vi "lamquenmatran.vi"() -> ()   [LabVIEW 2019]
uses:
  <vilib>/Analysis/Matrix/Datatypes/RealMatrix.ctl
  <vilib>/Platform/TimedLoop/XDataNode/timing_clust.ctl
  <vilib>/Platform/TimedLoop/XDataNode/nitl_modes.ctl
  <vilib>/Platform/TimedLoop/XDataNode/wakeup.ctl
  <vilib>/Analysis/Matrix/Numeric/Conversions/Matrix To Array - RM.vi
  <vilib>/imath/engines/lvmath2/RunTimeEngine/BuiltInFunctions/is_empty/NIMS_is_empty(GM).vi
  <instcachedir>/0/NIMS_is_empty(GM)_AF8F13F4B7FD436CB1855477E2504B8A.lvgen/NIMS_is_empty(GM)_AF8F13F4B7FD436CB1855477E2504B8A_004.vi
  <vilib>/imath/engines/lvmath2/RunTimeEngine/ArithmeticOperatorToken/NIMS_ArithmeticOperator_multmx(M,CV)-internal.vi
  <instcachedir>/0/NIMS_ArithmeticOperator_multmx(M,CV)-internal_2C55777844884EEDB828A940D397C7D0.lvgen/NIMS_ArithmeticOperator_multmx(M,CV)-internal_2C55777844884EEDB828A940D397C7D0_001.vi
  <vilib>/imathl/engines/lvmath/Functions/Error Handling/Create Error.vi
  <vilib>/imath/engines/lvmath2/RunTimeEngine/IndexRead/NIMS V(S).vi
  <instcachedir>/0/NIMS V(S)_0488751826AF41519A22953C041130DC.lvgen/NIMS V(S)_0488751826AF41519A22953C041130DC_000.vi
  <vilib>/imath/engines/lvmath2/RunTimeEngine/ArithmeticOperatorToken/NIMS_ArithmeticOperator_minus.vi
  <instcachedir>/0/NIMS_ArithmeticOperator_minus_12BFF9710EA5430A9EE87C5BC3F65186.lvgen/NIMS_ArithmeticOperator_minus_12BFF9710EA5430A9EE87C5BC3F65186_002.vi
  <vilib>/imath/engines/lvmath2/RunTimeEngine/ArithmeticOperatorToken/NIMS_ArithmeticOperator_plus.vi
  <instcachedir>/0/NIMS_ArithmeticOperator_plus_5C9385B0197D46E2B844C41E02F9EC39.lvgen/NIMS_ArithmeticOperator_plus_5C9385B0197D46E2B844C41E02F9EC39_003.vi
  <vilib>/imath/engines/lvmath2/RunTimeEngine/ErrorHandling/NIMS_Create Error From Enums.vi
  <vilib>/imath/engines/lvmath2/RunTimeEngine/RowToken/NIMS_RowToken_M_M.vi
  <instcachedir>/0/NIMS_RowToken_M_M_21FE36D058524603B8B587AC30FD72C2.lvgen/NIMS_RowToken_M_M_21FE36D058524603B8B587AC30FD72C2_004.vi
  <vilib>/imath/engines/lvmath2/RunTimeEngine/ArithmeticOperatorToken/NIMS_ArithmeticOperator_multmx(M,CV).vi
  <instcachedir>/0/NIMS_ArithmeticOperator_multmx(M,CV)_1D61EED49E1847F3B05DBB8EDD2FBF8F.lvgen/NIMS_ArithmeticOperator_multmx(M,CV)_1D61EED49E1847F3B05DBB8EDD2FBF8F_000.vi
  <vilib>/imath/engines/lvmath2/RunTimeEngine/IndexRead/NIMS M(S).vi
  <instcachedir>/0/NIMS M(S)_B826C018497E4940AE96BD27B540B6FB.lvgen/NIMS M(S)_B826C018497E4940AE96BD27B540B6FB_000.vi
  <vilib>/imath/engines/lvmath2/RunTimeEngine/VariableToken/NIMS_VariableToken_CondDefined.vi
  <instcachedir>/0/NIMS_VariableToken_CondDefined_30C3C94EAC01413DA882E848DEC89944.lvgen/NIMS_VariableToken_CondDefined_30C3C94EAC01413DA882E848DEC89944_001.vi
  <vilib>/Analysis/Matrix/Numeric/Conversions/Array To Matrix - RA2.vi
  <instcachedir>/0/NIMS_VariableToken_CondDefined_30C3C94EAC01413DA882E848DEC89944.lvgen/NIMS_VariableToken_CondDefined_30C3C94EAC01413DA882E848DEC89944_005.vi
  <vilib>/imath/engines/lvmath/Functions/Error Handling/MergeErrorsWrapper.vi
  <vilib>/imath/engines/lvmath2/RunTimeEngine/NodeEndStatement/NIMS_NodeEndStatement_Output.vi
  <instcachedir>/0/NIMS_NodeEndStatement_Output_53EC0D466D134D7ABD903AC30B43404B.lvgen/NIMS_NodeEndStatement_Output_53EC0D466D134D7ABD903AC30B43404B_002.vi
  <instcachedir>/0/NIMS_NodeEndStatement_Output_53EC0D466D134D7ABD903AC30B43404B.lvgen/NIMS_NodeEndStatement_Output_53EC0D466D134D7ABD903AC30B43404B_012.vi
  <instcachedir>/0/NIMS_NodeEndStatement_Output_53EC0D466D134D7ABD903AC30B43404B.lvgen/NIMS_NodeEndStatement_Output_53EC0D466D134D7ABD903AC30B43404B_001.vi
  <vilib>/imath/engines/lvmath2/RunTimeEngine/ErrorHandling/NIMS_Finalize Error.vi
  <vilib>/platform/TimedLoop/XDataNode/XDataNode.xnode
  <vilib>/Platform/TimedLoop/XDataNode/XDNodeRunTimeDep.lvlib
  <vilib>/Analysis/Matrix/NI_Matrix.lvlib
panel:
  out "b":dbl[][](array[numeric])
  out "c":dbl[][](array[numeric])
  out "m":dbl[][](array[numeric])
  out "a 2":dbl[][](array[numeric])
  out "Numeric":i32
  out "duty 2":T1
  out "K":dbl[][](array[numeric])
  out "Real Matrix 2":T1
  out "Real Matrix":T1
  out "e_k":T1 caption="Real Matrix"
  out "duty":T1 caption="Real Matrix"
  out "error out":errorcluster
  out "T":dbl
  in  "enable":bool
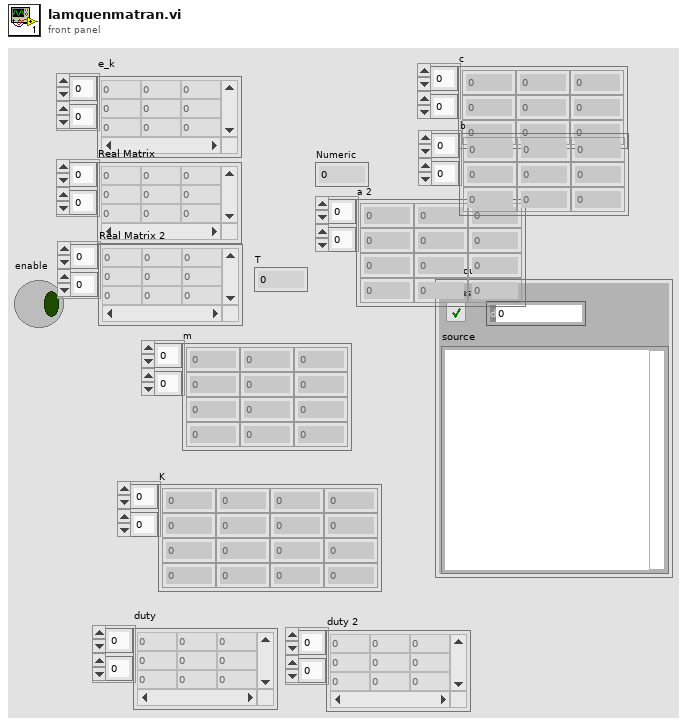
[diagram p1: front panel]
types:
  T1 = typedef "NI_Matrix.lvlib/RealMatrix.ctl" = dbl[][]
  T2 = typedef "XDNodeRunTimeDep.lvlib/timing_clust.ctl" = cluster{"Expected End [f-1]":u64, "Actual End [f-1]":u64, "Finished Late? [f-1]":bool, "Expected End [i-1]":u64, "Actual End [i-1]":u64, "Finished Late? [i-1]":bool, "Expected Start [i]":u64, "Actual Start [i]":u64, "Expected Start [f]":u64, "Actual Start [f]":u64, "Source Name":string, "Structure Name":string, "Period":i64, "Deadline":i64, "Offset":i64, "Start":i64, "Priority":i32, "Timeout":i32, "Mode":T3, "Wakeup Reason":T4, "Error":errorcluster, "Source Type":string, "Secondary Source Type":string, "Global End Time":u64, "Global Start Time":u64, "Frame Duration":u64, "Iteration Duration":u64, "Assigned CPU":i32, "I/O Scan Engine Mode":u32}
  T3 = typedef "XDNodeRunTimeDep.lvlib/nitl_modes.ctl" = enum32{"No Change", "Process missed periods, maintain original phase", "Discard missed periods, maintain original phase", "Process missed periods, ignore original phase", "Discard missed periods, ignore original phase"}
  T4 = typedef "XDNodeRunTimeDep.lvlib/wakeup.ctl" = enum32{"Normal", "Aborted", "Asynchronous wakeup", "Timing source error", "Timed loop error", "Timeout"}
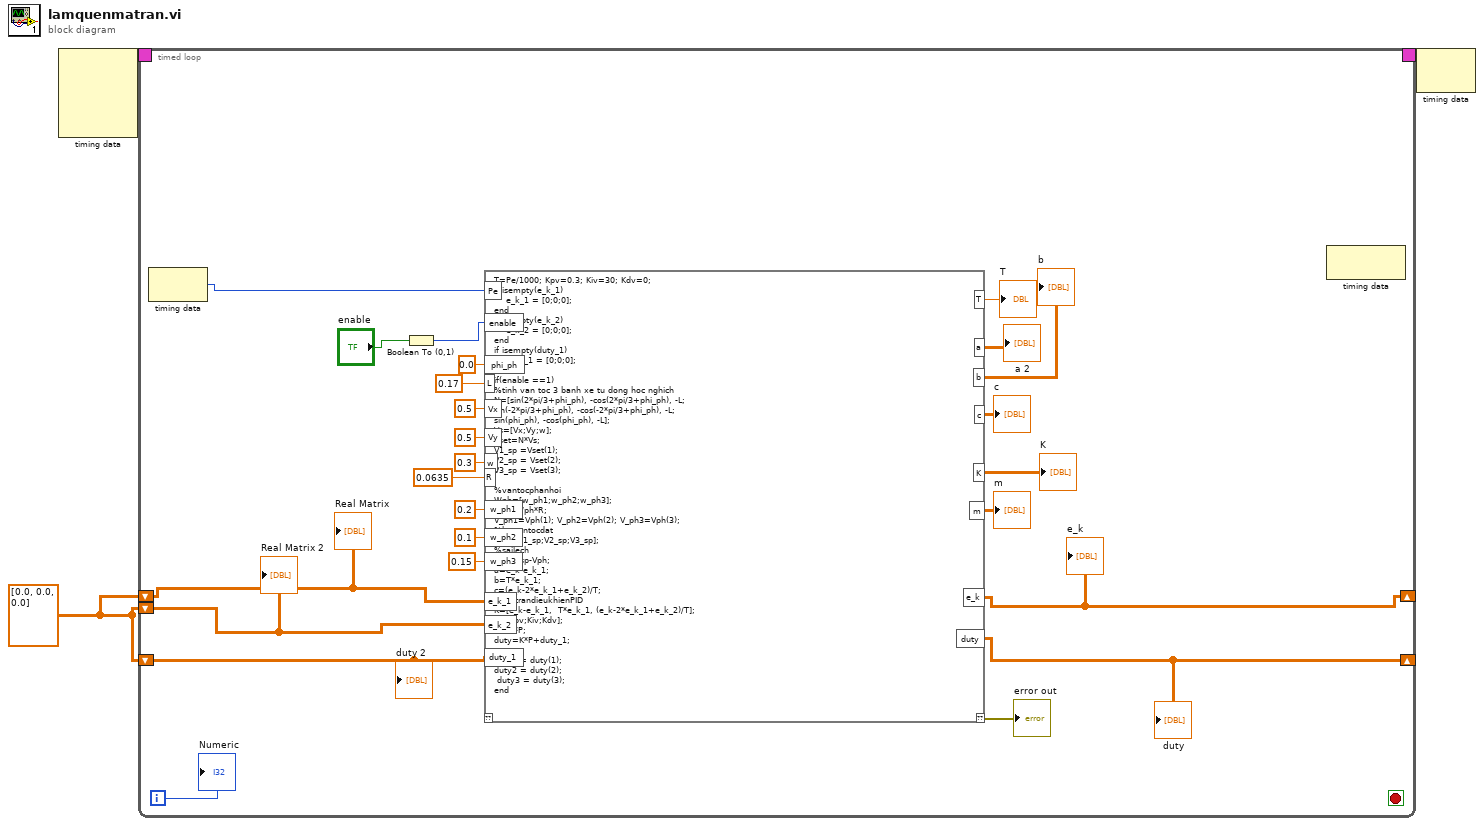
[diagram p0: block diagram]
diagram:
  w1 = T1 [[0.0], [0.0], [0.0]] ("e_k")
  n1 = node-c288() -> (w3:T2)  [unwired: 4 in]
  n2 = timed-loop {
    timing: w3 -> [_]
    timing-out: [_] -> w2
    shift-right: [w14] -> _
    shift-left: w1 -> [w13]
    shift-right: [w10] -> _
    shift-left: w1 -> [w12]
    shift-left: w1 -> [w11]
    i -> [w8]
    stop <- _ stop-if-true
    n3 = node-c288() -> (w28:i64)  [unwired: 1 in]
    n4 = Boolean To (0,1)(Boolean="enable") -> (0, 1=w26:i16)
    n5 = mathscript code="T=Pe/1000; Kpv=0.3; Kiv=30; Kdv=0;\nif isempty(e_k_1)\n    e_k_1 = [0;0;0]; \nend\nif isempty(e_k_2)\n    e_k_2 = [0;0;0]; \nend\nif isempty(duty_1)\n    duty_1 = [0;0;0]; \nend\nif(enable ==1)\n%tinh van toc 3 banh xe tu dong hoc nghich\nN=[sin(2*pi/3+phi_ph), -cos(2*pi/3+phi_ph), -L;\nsin(-2*pi/3+phi_ph), -cos(-2*pi/3+phi_ph), -L;\nsin(phi_ph), -cos(phi_ph), -L];\nVs=[Vx;Vy;w];\nVset=N*Vs;\nV1_sp =Vset(1);\nV2_sp = Vset(2);\nV3_sp = Vset(3);\n\n%vantocphanhoi\nWph=[w_ph1;w_ph2;w_ph3];\nVph=Wph*R;\nV_ph1=Vph(1); V_ph2=Vph(2); V_ph3=Vph(3);\n%locvantocdat\nVsp=[V1_sp;V2_sp;V3_sp];\n%sailech\ne_k=Vsp-Vph;\na=e_k-e_k_1;\nb=T*e_k_1;\nc=(e_k-2*e_k_1+e_k_2)/T;\n%matrandieukhienPID\nK=[e_k-e_k_1,  T*e_k_1, (e_k-2*e_k_1+e_k_2)/T];\nP=[Kpv;Kiv;Kdv];\nm=K*P;\nduty=K*P+duty_1;\n\nduty1 = duty(1);\nduty2 = duty(2);\n duty3 = duty(3);\nend"("Pe"=w28, "enable"=w26, "phi_ph"=0.0, "L"=0.17, "Vx"=0.5, "Vy"=0.5, "w"=0.3, "w_ph1"=0.2, "w_ph2"=0.1, "w_ph3"=0.15, "R"=0.0635, "e_k_1"=w12, "e_k_2"=w11, "duty_1"=w13) -> ("??"=→"error out":errorcluster, "T"=→"T":dbl, "e_k"=w10:T1, "duty"=w14:T1, "a"=→"a 2":dbl[][], "b"=→"b":dbl[][], "c"=→"c":dbl[][], "K"=→"K":dbl[][], "m"=→"m":dbl[][])  [unwired: 1 in]
    "duty" <- w14
    "e_k" <- w10
    n6 = node-c288() -> ()  [unwired: 1 in, 1 out]
    "Real Matrix" <- w12
    "Real Matrix 2" <- w11
    "duty 2" <- w13
    "Numeric" <- w8
  }
  n7 = node-c288(w2) -> ()  [unwired: 1 out]
